vi "load config data.vi"(8 "error in (no error)":errorcluster, 11 "FINE SIM Motion Axis in":refnum<class "FINE SIM Motion Axis.lvclass">) -> (0 "error out":errorcluster, 3 "FINE SIM Motion Axis out":refnum<class "FINE SIM Motion Axis.lvclass">)   [LabVIEW 2022 SP3, in "FINE SIM Motion Axis.lvclass"]
uses:
  FINE SIM Motion Axis.lvclass
  FINE SIM Motion Axis.lvclass/FINE SIM Motion Axis.ctl
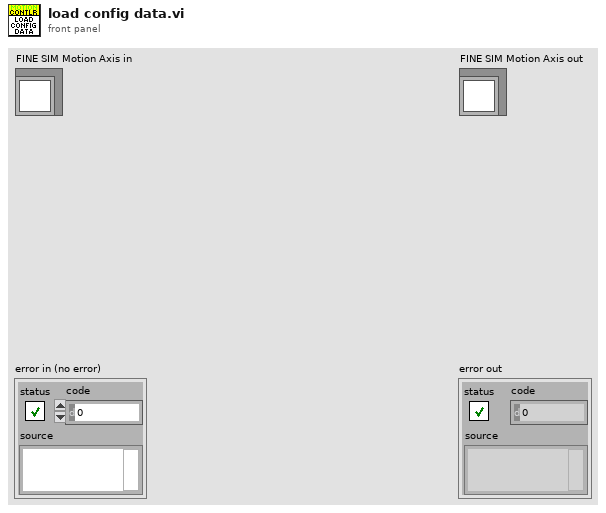
[diagram p1: front panel]
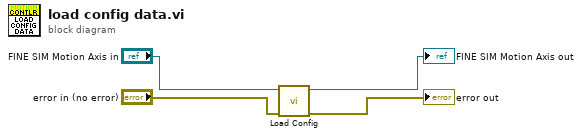
[diagram p0: block diagram]
diagram:
  n1 = call-dynamic "Load Config.vi"("error in (no error)"="error in (no error)", "Motion Controller in"="FINE SIM Motion Axis in") -> ("error out"=→"error out":errorcluster, "Motion Controller out"=→"FINE SIM Motion Axis out":refnum<class "FINE SIM Motion Axis.lvclass">)  [unwired: 8 in]
